vi "sample.vi"() -> ()   [LabVIEW 2013]
uses:
  <vilib>/Utility/file.llb/Write To Spreadsheet File (DBL).vi
panel:
  out "loops":i32
  out "Array":dbl[](array[numeric])
  out "error out":errorcluster
  out "VISA resource name out":refnum<visa-resource-name>
  in  "VISA resource name":refnum<visa-resource-name>="34405A"
  in  "error in (no error)":errorcluster
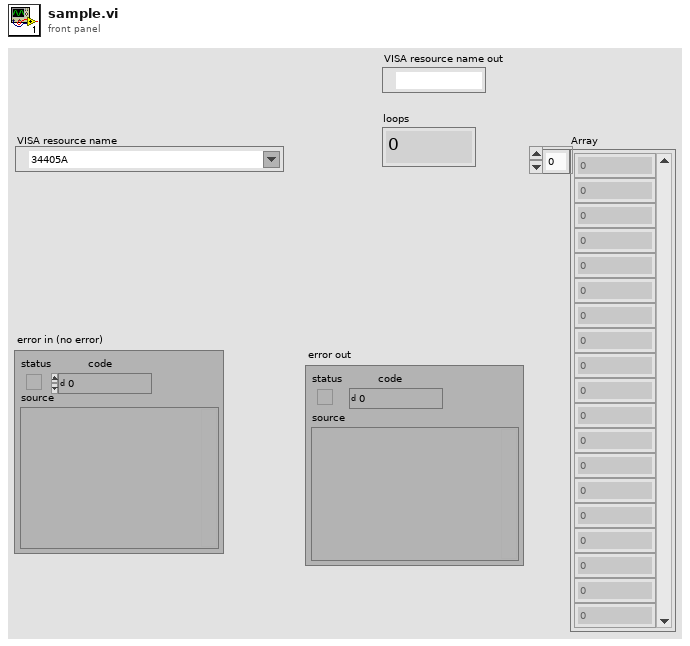
[diagram p1: front panel]
types:
  T1 = enum16{"DmmGetInfo", "DmmInit", "DmmOhms", "DmmDCvolts", "DmmACvolts", "DmmFreq", "DmmTemp", "DmmCap", "DmmAlarmHi", "DmmAlarmLow"}
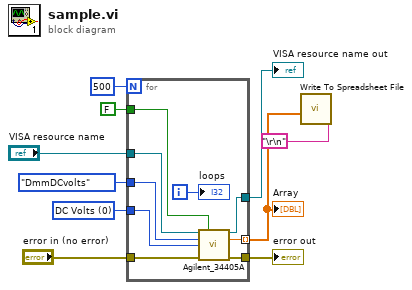
[diagram p0: block diagram]
diagram:
  w6 = u16 0 items=["DC Volts", "AC Volts", "DC Current", "AC Current", "2-Wire Resistance", "Frequency", "Temperature", "Capacitance", "Continuity", "Diode"] ("DMM Mode (0: DC Volts)")
  n1 = for {
    N: 500 -> [_]
    tunnel: "error in (no error)" -> [w19]
    tunnel: "VISA resource name" -> [w18]
    tunnel: T1."DmmDCvolts" ("Op") -> [w17]
    tunnel: FALSE ("Enable Auto Range (T:Enable)") -> [w16]
    tunnel: w6 -> [w15]
    tunnel: [w14] -> w5
    tunnel: [w13] -> w2 mode=indexing
    tunnel: [w12] -> w4
    i -> [w11]
    n2 = call "Agilent_34405A.vi"("VISA resource name"=w18, "Enable Auto Range (T:Enable)"=w16, "Op"=w17, "DMM Mode (0: DC Volts)"=w15, "error in (no error)"=w19) -> ("VISA resource name out"=w14:refnum<visa-resource-name>, "First data item"=w13:dbl, "error out"=w12:errorcluster)  [unwired: 5 in, 3 out]
    "loops" <- w11
  }
  "VISA resource name out" <- w5
  "error out" <- w4
  "Array" <- w2
  n3 = call-poly <vilib>:"Write To Spreadsheet File.vi"("delimiter (\\t)"="\r\n", "1D data"=w2) -> ()  [unwired: 6 in, 1 out]
